vi "log_raw_data.vi"(7 "G1 trigger in":bool, 8 "error in (no error)":errorcluster, 9 "Array":waveform(dbl)[](array[waveform]), 10 "AVI Path in":path, 11 "Refnum in":refnum<k34>) -> (0 "error out":errorcluster, 1 "AVI Path out":path, 2 "Acceleration Log Folder":path=path "/home/lvuser/Log/logfiles_deploy", 3 "Refnum out":refnum<k34>, 4 "AVI Path 3":path, 5 "G1 trigger out":bool)   [LabVIEW 2017]
uses:
  Globals/Global - All RT Loop Stop.vi
  Globals/Global - Configuration Options.vi
  UI Error Handlers/support/Logging/Logging.lvlib
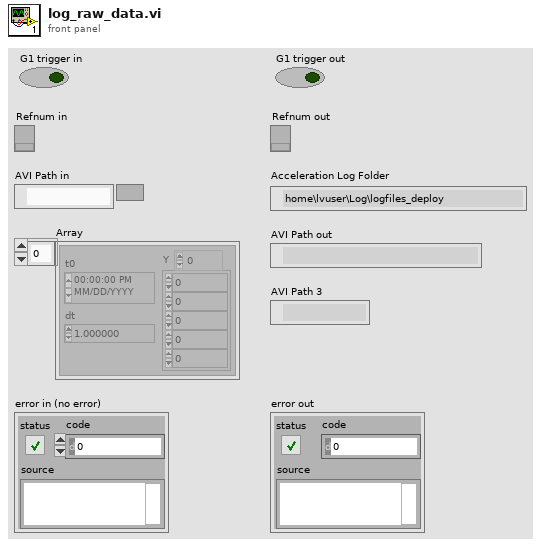
[diagram p1: front panel]
types:
  T1 = cluster{"Tool data":cluster{"Number of teeth":sgl}, "Cutting data":cluster{"rpm":sgl}, "Limits":cluster{"Magnitude threshold":sgl, "Tolerance":sgl}, "G1 status":cluster{"G1 trigger":bool}}
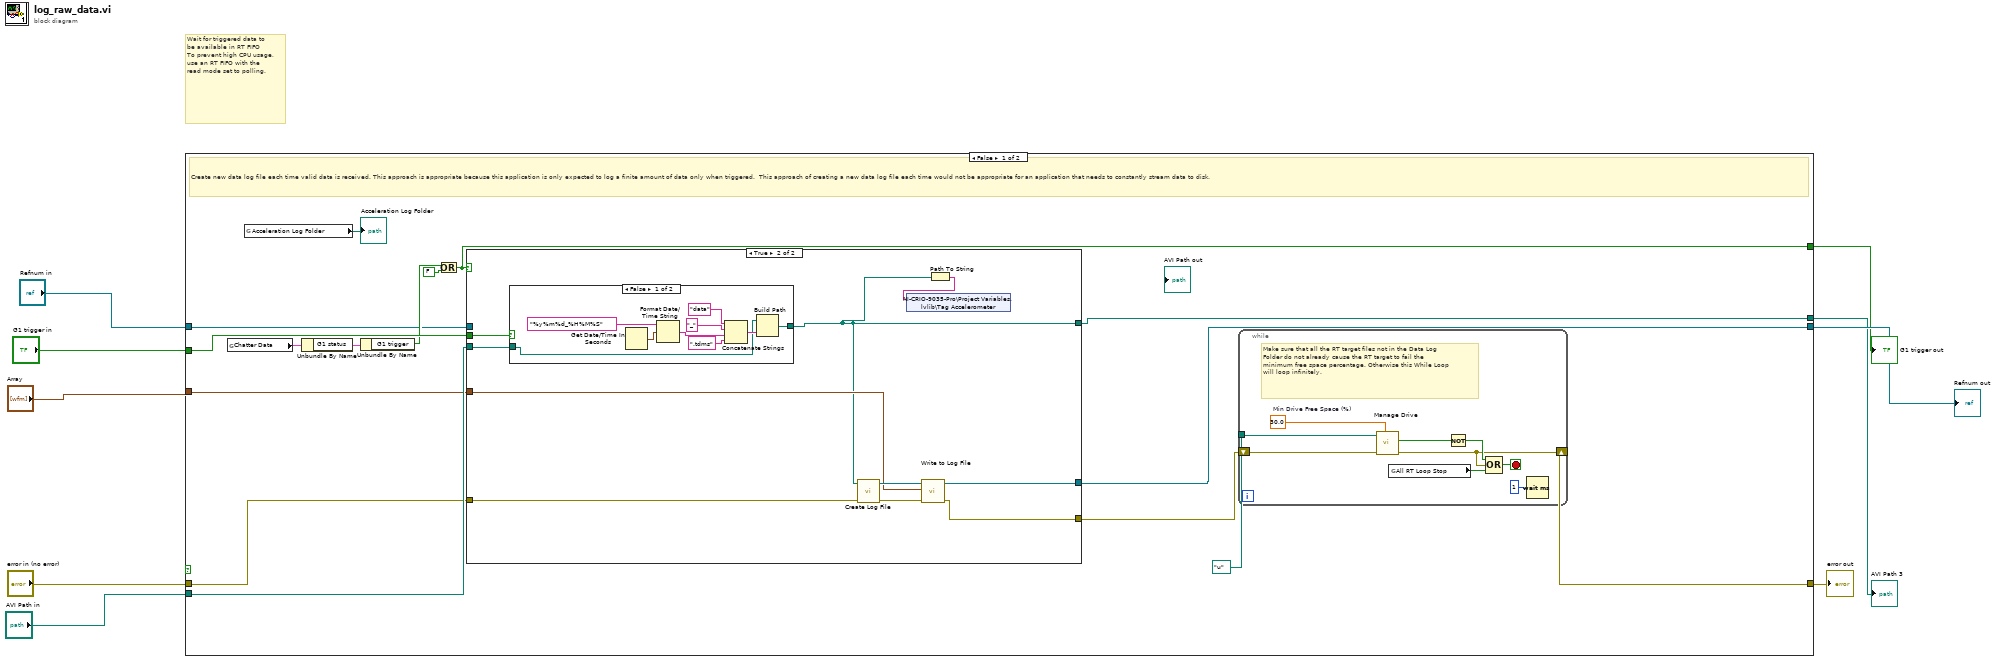
[diagram p0: block diagram]
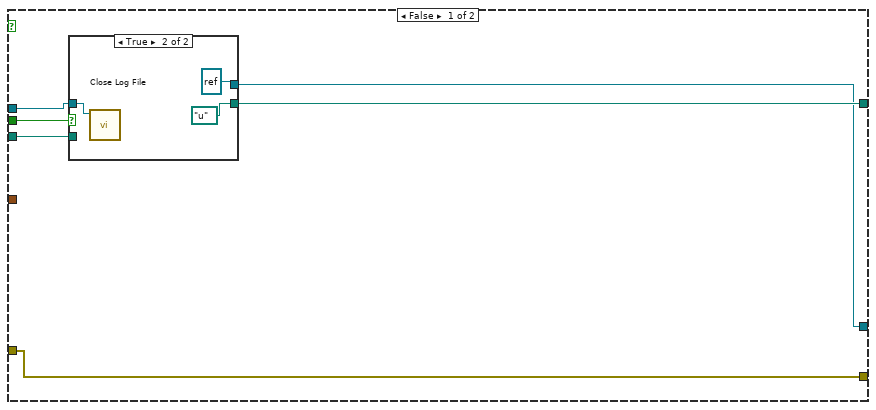
[diagram p2: hidden frame]
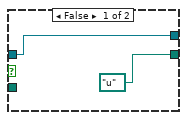
[diagram p3: hidden frame]
diagram:
  # "Wait for triggered data to be available in RT FIFO\nTo prevent high CPU usage, use an RT FIFO with the read mode set to polling."
  n1 = case shown="False" {
    selector: _ -> [_ _]
    tunnel: "Array" -> [w14 _]
    tunnel: "error in (no error)" -> [w12 w69]
    tunnel: [w15 w69] -> w1
    tunnel: [w10 w68] -> w2
    tunnel: "AVI Path in" -> [w21 w68]
    tunnel: [w18 w67] -> w4
    tunnel: "G1 trigger in" -> [w20 w67]
    tunnel: [w13 w66] -> w6
    tunnel: "Refnum in" -> [w16 w66]
    frame False {
      # "Create new data log file each time valid data is received. This approach is appropriate because this application is only expected to log a finite amount of data only when triggered.  This approach of creating a new data log file each time would not be appropriate for an application that needs to constantly stream data to disk."
      n2 = global read "Global - Configuration Options.vi" "Chatter Data"() -> (w23:T1)
      n3 = global read "Global - Configuration Options.vi" "Acceleration Log Folder"() -> (→"Acceleration Log Folder":path)
      n4 = Unbundle By Name(w23) -> ("G1 status"=w22:cluster{"G1 trigger":bool})
      n5 = Unbundle By Name(w22) -> ("G1 trigger"=w19:bool)
      n6 = Or(x=w19, y=FALSE) -> (x .or. y?=w18:bool)
      n7 = case shown="True" w18 {
        tunnel: w21 -> [w28 w46]
        tunnel: [w31 w40] -> w10
        tunnel: w20 -> [w29 w45]
        tunnel: w16 -> [w30 _]
        tunnel: w14 -> [_ w42]
        tunnel: [w27 w39] -> w13
        tunnel: w12 -> [w26 w38]
        tunnel: [w26 w37] -> w11
        frame False {
          n8 = case shown="True" w29 {
            tunnel: [path "u:/" ("AVI Path") path "u:/" ("AVI Path")] -> w31
            tunnel: w30 -> [w32 w35]
            tunnel: w28 -> [_ _]
            tunnel: [w32 refnum<k34> refnum ("Log File out")] -> w27
            frame False {
            }
            frame True {
              n9 = call "Close Log File.vi"("tdms file"=w35) -> ()  [unwired: 10 in, 1 out]
            }
          }
        }
        frame True {
          n10 = case shown="False" w45 {
            tunnel: w46 -> [w48 w56]
            tunnel: [w47 w56] -> w40
            frame False {
              n11 = Get Date/Time In Seconds() -> (seconds since 1Jan1904=w51:timestamp)
              n12 = Format Date/Time String(time format string (%c)="%y%m%d_%H%M%S", seconds (now)=w51) -> (date/time string=w54:string)  [unwired: 1 out]
              n13 = Concatenate Strings("data" ("string"), "_" ("string"), w54, ".tdms" ("string")) -> (w49:string)
              n14 = Build Path(base path=w48, name or relative path=w49) -> (appended path=w47:path)
            }
            frame True {
            }
          }
          n15 = call "Create Log File.vi"("error in (no error)"=w38, "Acceleration Exceeded Log Folder"=w40) -> ("error out"=w44:errorcluster, "Log File out"=w43:refnum<k34>)  [unwired: 8 in]
          n16 = call "Write to Log File.vi"("error in (no error)"=w44, "Array of Waveforms"=w42, "Log File in"=w43) -> ("error out"=w37:errorcluster, "Log File out"=w39:refnum<k34>)  [unwired: 7 in]
          n17 = Path To String(path=w40) -> (string=w41:string)
          n18 = shared-variable "NI-CRIO-9035-Pro\\Project Variables.lvlib\\Tag Accelerometer"(w41) -> ()  [unwired: 1 in, 1 out]
        }
      }
      n19 = while {
        shift-right: [w60] -> w15
        shift-left: w11 -> [w61]
        tunnel: path "u:/" ("AVI Path") -> [w58]
        stop <- w65 stop-if-true
        w59 = 30.0  # Min Drive Free Space (%)
        # "Make sure that all the RT target files not in the Data Log Folder do not already cause the RT target to fail the minimum free space percentage. Otherwise this While Loop will loop infinitely."
        n20 = call "Manage Drive.vi"("Min Drive Free Space (%)"=w59, "error in"=w61, "Data Folder"=w58) -> ("error out"=w60:errorcluster, "Drive Space Below Limit"=w57:bool)  [unwired: 7 in]
        n21 = global read "Global - All RT Loop Stop.vi" "All RT Loop Stop"() -> (w62:bool)
        n22 = Not(x=w57) -> (.not. x?=w64:bool)
        n23 = Compound Arithmetic op=OR(w64, w60, w62) -> (w65:bool)
        n24 = Wait (ms)(milliseconds to wait=u32 1) -> ()  [unwired: 1 out]
      }
    }
    frame True {
      # "Timed out - No data"
    }
  }
  "Refnum out" <- w6
  "G1 trigger out" <- w4
  "AVI Path 3" <- w2
  "error out" <- w1
